vi "demo_data_out.vi"(8 "error in (no error)":errorcluster) -> (0 "error out":errorcluster, 3 "camera data string":string)   [LabVIEW 2013, in "Camera.lvclass"]
uses:
  Camera.lvclass
  Experiment/Globals.vi
  TCP_IP/TCP_IP.lvclass
panel:
  out "Intensity Graph":u16[][](graph)
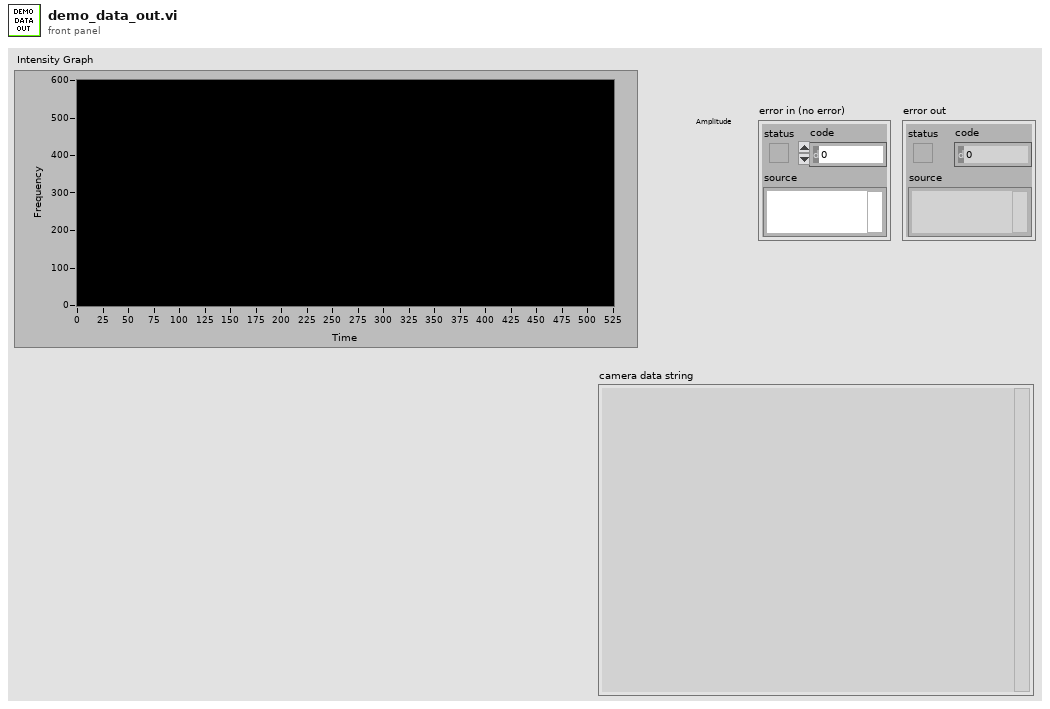
[diagram p1: front panel]
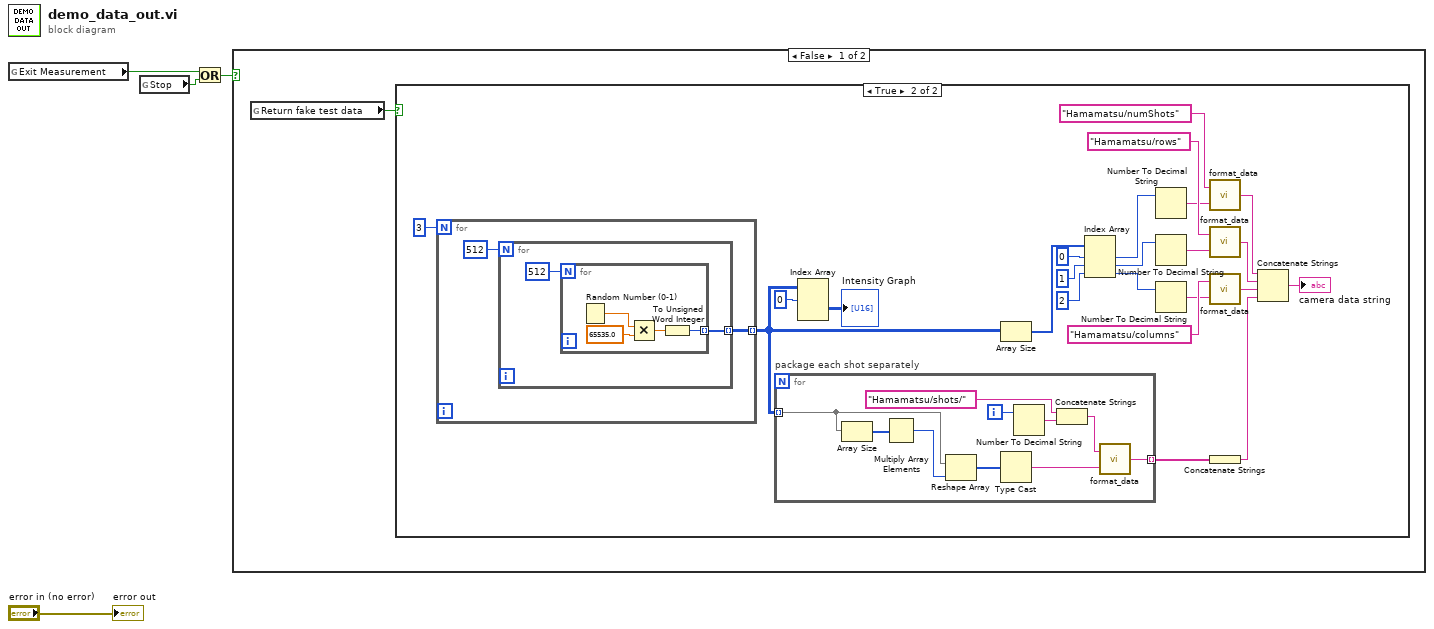
[diagram p0: block diagram]
diagram:
  n1 = global read "Globals.vi" "Exit Measurement"() -> (w3:bool)
  n2 = global read "Globals.vi" "Stop"() -> (w2:bool)
  n3 = Or(x=w3, y=w2) -> (x .or. y?=w1:bool)
  n4 = case shown="False" w1 {
    frame False {
      n5 = global read "Globals.vi" "Return fake test data"() -> (w5:bool)
      n6 = case shown="True" w5 {
        frame False {
        }
        frame True {
          n7 = for {
            N: 3 -> [_]
            tunnel: [w29] -> w9 mode=indexing
            n8 = for {
              N: 512 -> [_]
              tunnel: [w31] -> w29 mode=indexing
              n9 = for {
                N: 512 -> [_]
                tunnel: [w33] -> w31 mode=indexing
                n10 = Random Number (0-1)() -> (number: 0 to 1=w36:dbl)
                n11 = Multiply(x=w36, y=65535.0) -> (x*y=w34:dbl)
                n12 = To Unsigned Word Integer(number=w34) -> (unsigned 16bit integer=w33:u16)
              }
            }
          }
          n13 = for "package each shot separately" {
            tunnel: w9 -> [w44] mode=indexing
            tunnel: [w39] -> w12 mode=indexing
            i -> [w42]
            n14 = Array Size(array=w44) -> (size(s)=w46:i32[])
            n15 = Multiply Array Elements(1:w46) -> (0:w45:i32)
            n16 = Reshape Array(w44, w45) -> (w38:u16[])
            n17 = Type Cast(x=w38) -> (*(type *) &x=w37:string)  [unwired: 1 in]
            n18 = Number To Decimal String(number=w42) -> (decimal integer string=w41:string)  [unwired: 1 in]
            n19 = Concatenate Strings("Hamamatsu/shots/" ("name"), w41) -> (w40:string)
            n20 = call "format_data.vi"("data"=w37, "name"=w40) -> ("concatenated string"=w39:string)
          }
          n21 = Index Array(array=w9, index (dim 0)=0 ("index (page)")) -> (element=→"Intensity Graph":u16[][])  [unwired: 2 in]
          n22 = Array Size(array=w9) -> (size(s)=w25:i32[])
          n23 = Index Array(array=w25, index #1=0 ("index"), index #2=1 ("index"), index #3=2 ("index")) -> (element #1=w20:i32, element #2=w19:i32, element #3=w16:i32)
          n24 = Number To Decimal String(number=w20) -> (decimal integer string=w21:string)  [unwired: 1 in]
          n25 = Number To Decimal String(number=w19) -> (decimal integer string=w18:string)  [unwired: 1 in]
          n26 = Number To Decimal String(number=w16) -> (decimal integer string=w17:string)  [unwired: 1 in]
          n27 = call "format_data.vi"("data"=w21, "name"="Hamamatsu/numShots") -> ("concatenated string"=w15:string)
          n28 = call "format_data.vi"("data"=w18, "name"="Hamamatsu/rows") -> ("concatenated string"=w14:string)
          n29 = call "format_data.vi"("data"=w17, "name"="Hamamatsu/columns") -> ("concatenated string"=w13:string)
          n30 = Concatenate Strings(w12) -> (w11:string)
          n31 = Concatenate Strings(w15, w14, w13, w11) -> (→"camera data string":string)
        }
      }
    }
    frame True {
    }
  }
  "error out" <- "error in (no error)"
